vi "DHE_GatherHdrInfo.vi"(9 "link info":string, 10 "ctrl info":string, 11 "DHE_DBSRef":T1) -> ()   [LabVIEW 2016]
uses:
  DBSHAND/private/vis/DatabaseHand_RefNum.ctl
  DBSHAND/private/vis/DatabaseHand_Element_Set(2DArr).vi
  DBSHAND/private/vis/DatabaseHand_Element_Set(string).vi
  DBSHAND/private/vis/DatabaseHand_Element_Get(2DArr).vi
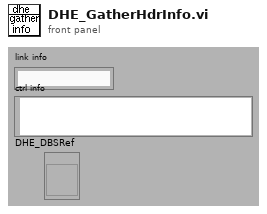
[diagram p1: front panel]
types:
  T1 = typedef "DatabaseHand_RefNum.ctl" = refnum<vi>
  T2 = enum16{"read from file", "clear", "get all", "set all"}
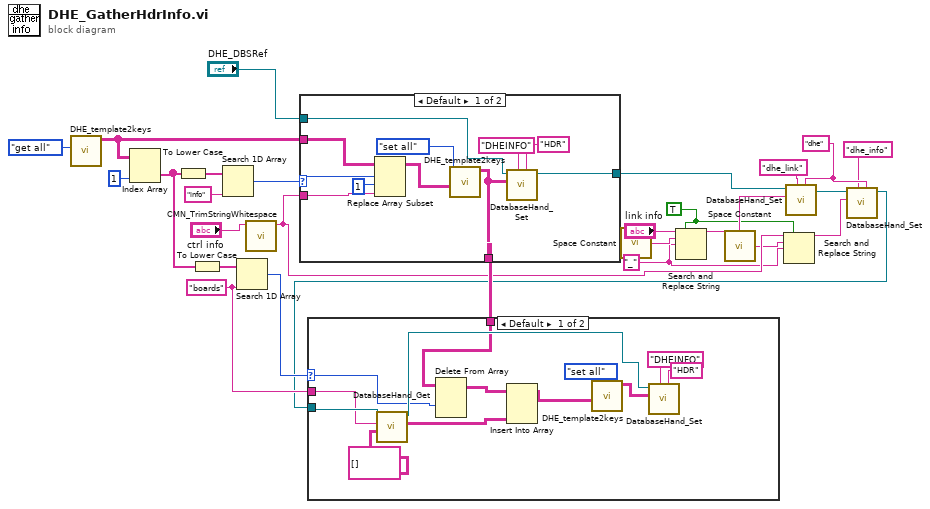
[diagram p0: block diagram]
diagram:
  w4 = "_" ("replace string (\"\")")
  w2 = TRUE ("replace all? (F)")
  w9 = "dhe" ("group")
  w17 = "boards" ("element")
  n1 = call "DHE_template2keys.vi"("Action"=T2."get all") -> ("HdrInfo"=w23:string[][])  [unwired: 3 in, 7 out]
  n2 = Index Array(array=w23, index (col)=1 ("disabled index (col)")) -> (element=w20:string[])  [unwired: 1 in]
  n3 = To Lower Case(string=w20) -> (all lower case string=w22:string[])
  n4 = To Lower Case(string=w20) -> (all lower case string=w21:string[])
  n5 = Search 1D Array(1D array=w22, element="info") -> (index of element=w24:i32)  [unwired: 1 out]
  n6 = Search 1D Array(1D array=w21, element=w17) -> (index of element=w19:i32)  [unwired: 1 out]
  n7 = call "CMN_TrimStringWhitespace.vi"("string"="ctrl info") -> ("trimmed string"=w6:string)  [unwired: 1 in, 8 out]
  n8 = case shown="Default" w24 {
    selector: w24 -> [w37 _]
    tunnel: w23 -> [w38 w40]
    tunnel: [w31 w40] -> w18
    tunnel: "DHE_DBSRef" -> [w30 w39]
    tunnel: w6 -> [w29 _]
    tunnel: [w28 w39] -> w1
    frame Default {
      n9 = Replace Array Subset(array=w38, new element=w29, index (row)=w37, index (col)=1 ("disabled index (col)")) -> (w35:string[][])
      n10 = call "DHE_template2keys.vi"("HdrInfo In"=w35, "Action"=T2."set all") -> ("HdrInfo"=w31:string[][])  [unwired: 2 in, 7 out]
      n11 = call-poly "DatabaseHand_Set.vi"("group"="HDR", "name"="DHEINFO", "value"=w31, "Database RefNum in"=w30) -> ("Database RefNum out"=w28:T1)  [unwired: 4 in, 3 out]
    }
    frame ..-1 {
    }
  }
  n12 = call <vilib>:"Space Constant.vi"() -> ("String"=w13:string)
  n13 = Search and Replace String(replace all?=w2, input string="link info", search string=w13, replace string=w4) -> (result string=w12:string)  [unwired: 1 in, 6 out]
  n14 = call <vilib>:"Space Constant.vi"() -> ("String"=w5:string)
  n15 = Search and Replace String(replace all?=w2, input string=w6, search string=w5, replace string=w4) -> (result string=w3:string)  [unwired: 2 in, 5 out]
  n16 = call-poly "DatabaseHand_Set.vi"("group"=w9, "name"="dhe_link", "value"=w12, "Database RefNum in"=w1) -> ("Database RefNum out"=w11:T1)  [unwired: 4 in, 3 out]
  n17 = call-poly "DatabaseHand_Set.vi"("group"=w9, "name"="dhe_info", "value"=w3, "Database RefNum in"=w11) -> ("Database RefNum out"=w10:T1)  [unwired: 4 in, 3 out]
  n18 = case shown="Default" w19 {
    selector: w19 -> [w41 _]
    tunnel: w18 -> [w44 _]
    tunnel: w10 -> [w49 _]
    tunnel: w17 -> [w48 _]
    frame Default {
      n19 = call-poly "DatabaseHand_Get.vi"("default value"=string[][] [], "name"=w48, "Database RefNum in"=w49) -> ("value"=w42:string[][], "Database RefNum out"=w45:T1)  [unwired: 2 in, 5 out]
      n20 = Delete From Array(array=w44, index (row)=w41) -> (array with subset deleted=w43:string[][])  [unwired: 2 in, 1 out]
      n21 = Insert Into Array(array=w43, new element=w42) -> (w46:string[][])  [unwired: 2 in]
      n22 = call "DHE_template2keys.vi"("HdrInfo In"=w46, "Action"=T2."set all") -> ("HdrInfo"=w52:string[][])  [unwired: 2 in, 7 out]
      n23 = call-poly "DatabaseHand_Set.vi"("group"="HDR", "name"="DHEINFO", "value"=w52, "Database RefNum in"=w45) -> ()  [unwired: 4 in, 4 out]
    }
    frame ..-1 {
    }
  }
